vi "LOOP.vi"(4 "error in (no error)":errorcluster, 5 "LOOP":i32(ring) items=["I", "V"], 7 "connection ID":refnum<k5>) -> (0 "error out":errorcluster, 3 "connection ID out":refnum<k5>)   [LabVIEW 2025, in "CAENels FAST-PS.lvlib"]
doc: "The LOOP command can be used in order to select the mode of loop control of the FAST-PS unit. There are two possible modes of operation:\n- I for Constant Current (c.c.) mode and \n- V for Constant Voltage (c.v.) mode."
uses:
  CAENels FAST-PS.lvlib
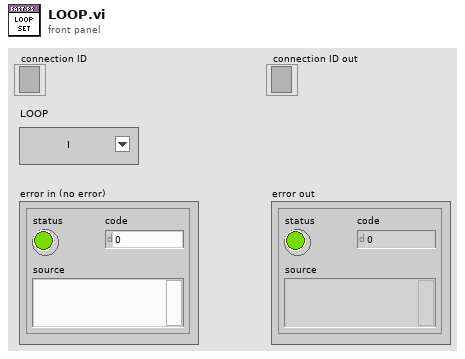
[diagram p1: front panel]
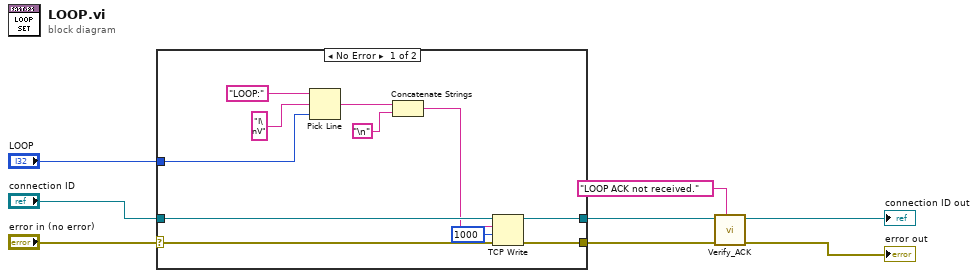
[diagram p0: block diagram]
diagram:
  n1 = case shown="No Error" "error in (no error)" {
    selector: "error in (no error)" -> [w19 w21]
    tunnel: [w18 w21] -> w5
    tunnel: [w17 w20] -> w3
    tunnel: "connection ID" -> [w16 w20]
    tunnel: "LOOP" -> [w13 _]
    frame No Error {
      n2 = Pick Line(string ("")="LOOP:", multi-line string="I\nV" ("string (\"\")"), line index=w13) -> (output string=w12:string)
      n3 = Concatenate Strings(w12, "\n") -> (w10:string)
      n4 = TCP Write(connection ID=w16, data in=w10, error in (no error)=w19, 9:1000 ("timeout ms (25000)")) -> (connection ID out=w17:refnum<k5>, error out=w18:errorcluster)  [unwired: 1 out]
    }
    frame Error {
    }
  }
  n5 = call "Verify_ACK.vi"("error code description"="LOOP ACK not received.", "error in (no error)"=w5, "connection ID"=w3) -> ("error out"=→"error out":errorcluster, "connection ID out"=→"connection ID out":refnum<k5>)  [unwired: 5 in]
